vi "Store Calibration Coefficients.vi"(0 "Calibration Coefficients":T1[](array[typedef]) {"Elapsed Time" format="%<%H:%M:%S>t"; "zero_utc" format="%x"; "cal_utc" format="%x"; "Pump Flow Rate" format="%0d"; "Number of Zeroes" format="%0d"; "V2C" format="%0d"; "C2V" format="%0d"; "duration" format="%<%H:%M:%S>t"; "DAC" format="%03x"; "mI" format="%.3g"; "V_(RA,15mA)" format="%0.4f"; "V_(RA,5mA)" format="%0.4f"; "Chamber Temp" format="%.1f"; "Humidity" format="%.1f"}, 1 "Zero_Humidity":dbl format="%.2f", 2 "Zero_Temperature":dbl format="%.2f", 3 "supporting caldata":string[][](array[string])) -> ()   [LabVIEW 2016]
uses:
  Controls/Calibration Coefficients.ctl
  Miscellaneous/Globals.vi
  <vilib>/Utility/file.llb/Write To Spreadsheet File (string).vi
panel:
  in  "Logfile":path=path "calibration_log.csv"
  out "Spreadsheet Out":string[][](array[string])
  in  "Calfile":path=path "~last_calibration.csv"
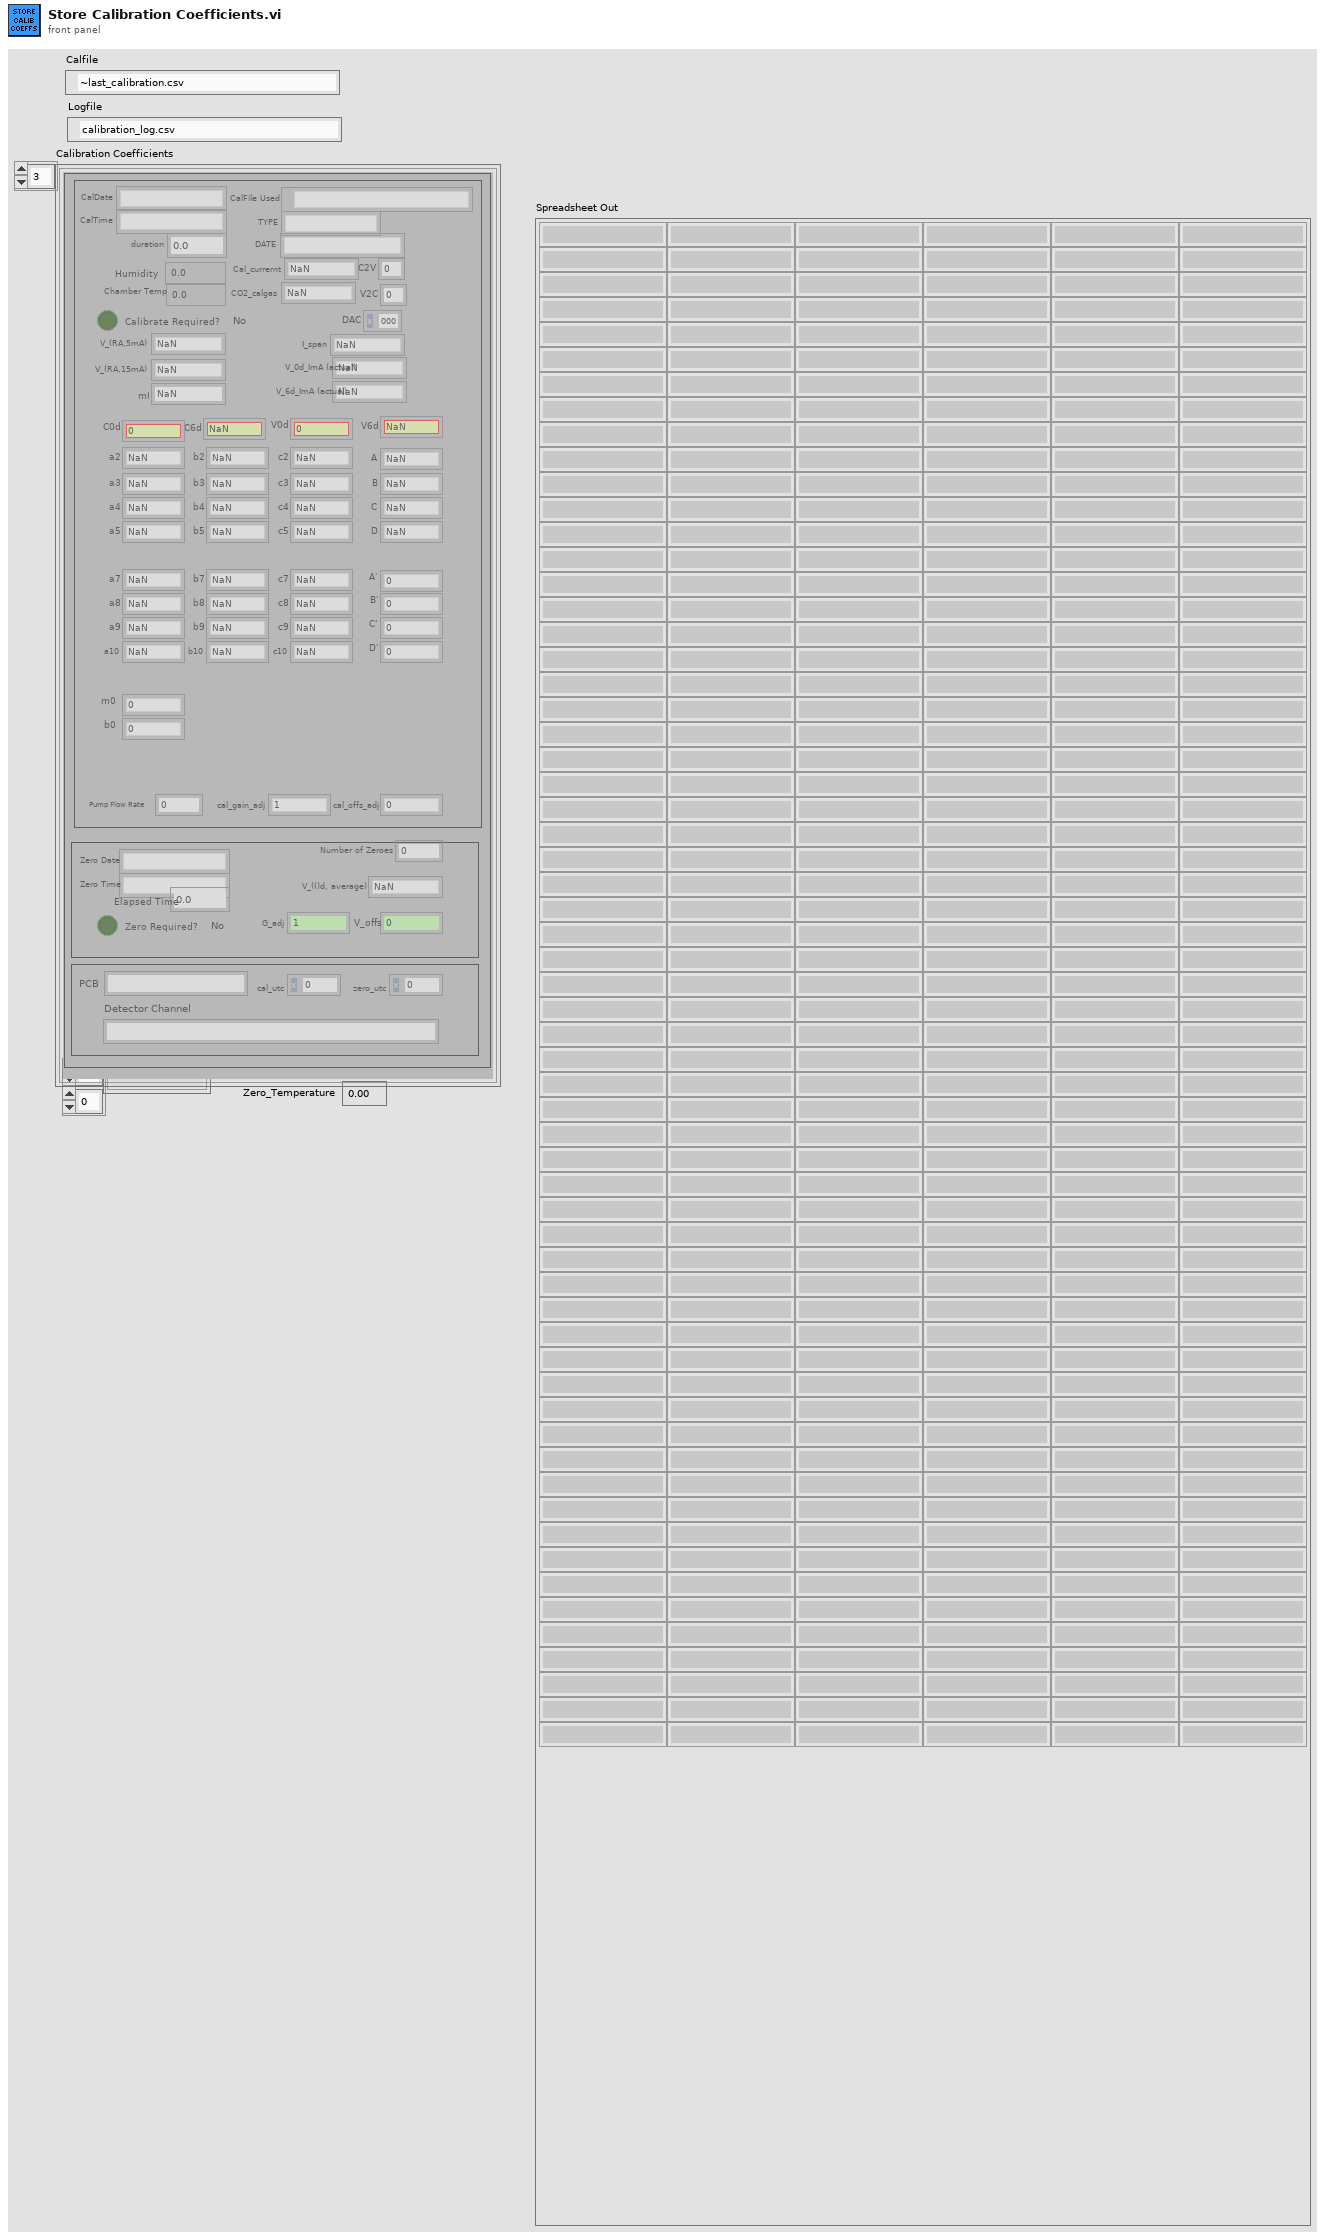
[diagram p1: front panel]
types:
  T1 = typedef "Calibration Coefficients.ctl" = cluster{"CalFile Used":path, "TYPE":string, "DATE":string, "Humidity":sgl, "Chamber Temp":dbl, "CO2_calgas":dbl, "V_(RA,5mA)":dbl, "V_(RA,15mA)":dbl, "mI":dbl, "V_0d_ImA (actual)":dbl, "V_6d_ImA (actual)":dbl, "I_span":dbl, "DAC":u16, "A":dbl, "B":dbl, "C":dbl, "D":dbl, "V6d":dbl, "A'":dbl, "B'":dbl, "C'":dbl, "D'":dbl, "V0d":dbl, "CalDate":string, "CalTime":string, "duration":dbl, "Detector Channel":string, "a2":dbl, "a3":dbl, "a4":dbl, "a5":dbl, "b2":dbl, "c2":dbl, "b3":dbl, "c3":dbl, "b4":dbl, "c4":dbl, "b5":dbl, "c5":dbl, "a7":dbl, "a8":dbl, "a9":dbl, "a10":dbl, "b7":dbl, "b8":dbl, "b9":dbl, "b10":dbl, "c7":dbl, "c8":dbl, "c9":dbl, "c10":dbl, "cal_offs_adj":dbl, "cal_gain_adj":dbl, "C6d":dbl, "C0d":dbl, "Cal_currernt":dbl, "C2V":u16, "V2C":u16, "Zero Date":string, "Zero Time":string, "Number of Zeroes":u16, "V_(()d, average)":dbl, "V_offs ":dbl, "G_adj":dbl, "Pump Flow Rate":u16, "Zero Required? ":bool, "Calibrate Required?":bool, "cal_utc":dbl, "zero_utc":dbl, "Elapsed Time":dbl, "PCB":string, "m0":dbl, "b0":dbl}
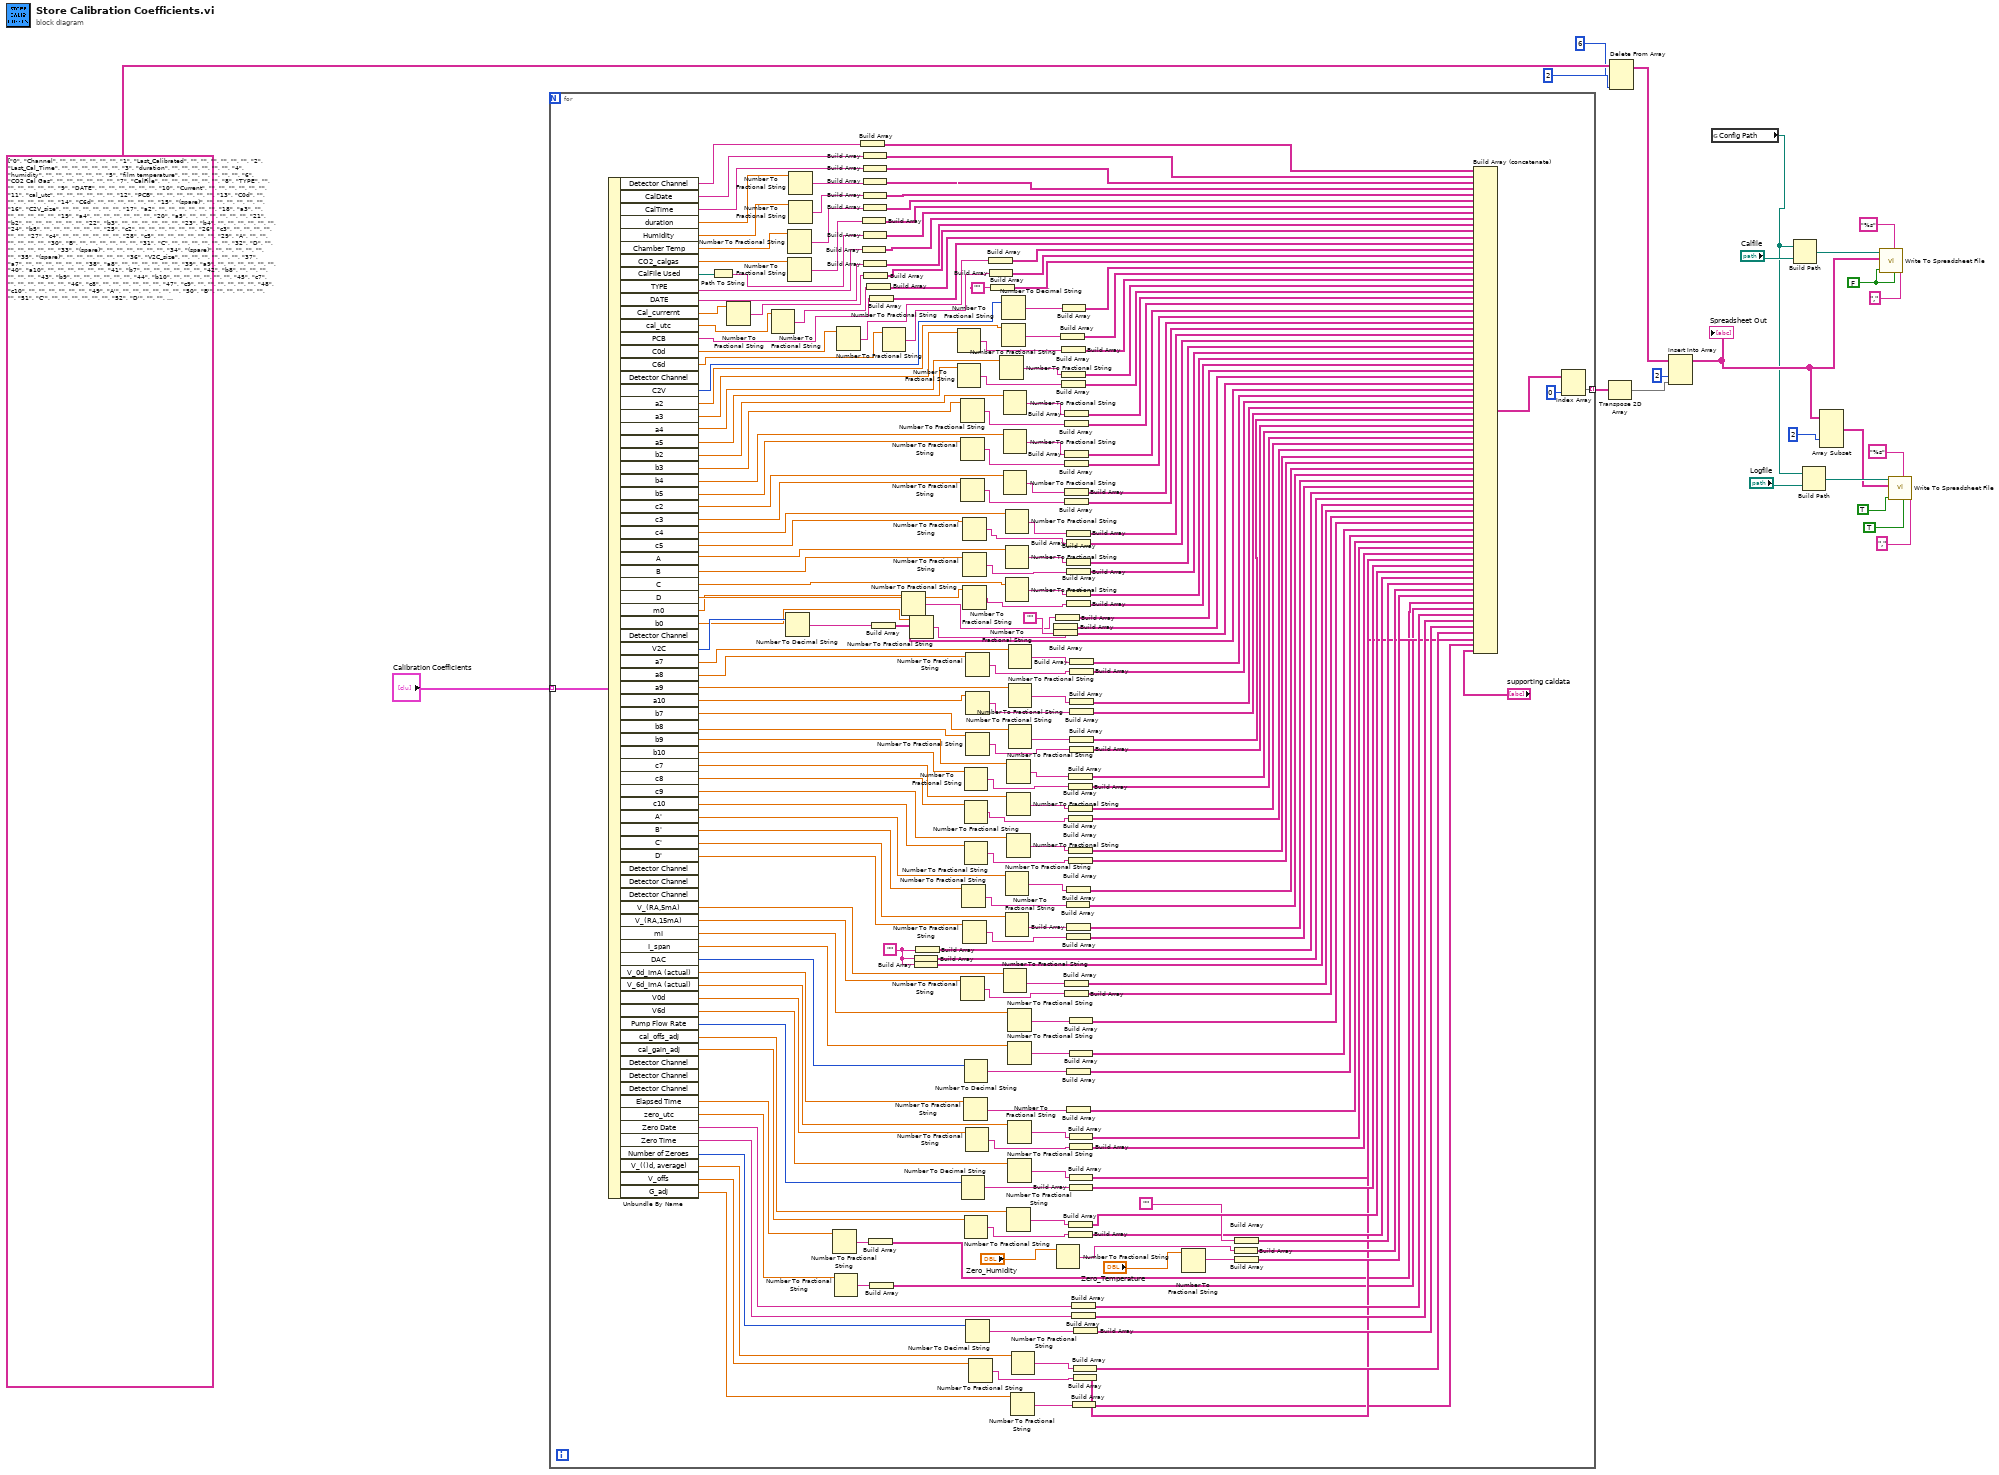
[diagram p0: block diagram]
diagram:
  w20 = FALSE ("transpose (no:F)")
  n1 = for {
    tunnel: [w166] -> w8 mode=indexing
    tunnel: "Calibration Coefficients" -> [w50] mode=indexing
    w87 = ""
    n2 = Unbundle By Name(w50) -> ("Detector Channel"=w55:string, "CalDate"=w249:string, "CalTime"=w248:string, "duration"=w246:dbl, "Humidity"=w163:sgl, "Chamber Temp"=w162:dbl, "CO2_calgas"=w157:dbl, "CalFile Used"=w155:path, "TYPE"=w153:string, "DATE"=w154:string, "Cal_currernt"=w44:dbl, "cal_utc"=w30:dbl, "PCB"=w28:string, "C0d"=w40:dbl, "C6d"=w39:dbl, "C2V"=w147:u16, "a2"=w145:dbl, "a3"=w144:dbl, "a4"=w143:dbl, "a5"=w142:dbl, "b2"=w141:dbl, "b3"=w140:dbl, "b4"=w139:dbl, "b5"=w138:dbl, "c2"=w137:dbl, "c3"=w136:dbl, "c4"=w135:dbl, "c5"=w134:dbl, "A"=w133:dbl, "B"=w132:dbl, "C"=w131:dbl, "D"=w130:dbl, "m0"=w27:dbl, "b0"=w26:dbl, "V2C"=w121:u16, "a7"=w124:dbl, "a8"=w123:dbl, "a9"=w114:dbl, "a10"=w113:dbl, "b7"=w112:dbl, "b8"=w111:dbl, "b9"=w110:dbl, "b10"=w109:dbl, "c7"=w108:dbl, "c8"=w107:dbl, "c9"=w106:dbl, "c10"=w105:dbl, "A'"=w103:dbl, "B'"=w102:dbl, "C'"=w101:dbl, "D'"=w100:dbl, "V_(RA,5mA)"=w99:dbl, "V_(RA,15mA)"=w98:dbl, "mI"=w97:dbl, "I_span"=w96:dbl, "DAC"=w90:u16, "V_0d_ImA (actual)"=w95:dbl, "V_6d_ImA (actual)"=w93:dbl, "V0d"=w92:dbl, "V6d"=w91:dbl, "Pump Flow Rate"=w89:u16, "cal_offs_adj"=w79:dbl, "cal_gain_adj"=w78:dbl, "Elapsed Time"=w42:dbl, "zero_utc"=w45:dbl, "Zero Date"=w71:string, "Zero Time"=w70:string, "Number of Zeroes"=w73:u16, "V_(()d, average)"=w68:dbl, "V_offs"=w67:dbl, "G_adj"=w66:dbl)  [unwired: 8 out]
    n3 = Path To String(path=w155) -> (string=w152:string)
    n4 = Number To Fractional String(number=w44) -> (F-format string=w31:string)  [unwired: 3 in]
    n5 = Number To Fractional String(number=w30) -> (F-format string=w29:string)  [unwired: 3 in]
    n6 = Number To Decimal String(number=w121) -> (decimal integer string=w122:string)  [unwired: 1 in]
    n7 = Number To Fractional String(number=w162) -> (F-format string=w160:string)  [unwired: 3 in]
    n8 = Number To Fractional String(number=w157) -> (F-format string=w156:string)  [unwired: 3 in]
    n9 = Number To Fractional String(number=w246) -> (F-format string=w245:string)  [unwired: 3 in]
    n10 = Number To Fractional String(number=w163) -> (F-format string=w161:string)  [unwired: 3 in]
    n11 = Number To Fractional String(number=w42) -> (F-format string=w43:string)  [unwired: 3 in]
    n12 = Number To Fractional String(number=w45) -> (F-format string=w47:string)  [unwired: 3 in]
    n13 = Number To Fractional String(number=w40) -> (F-format string=w37:string)  [unwired: 3 in]
    n14 = Build Array(w55) -> (w54:string[])
    n15 = Build Array(w156) -> (w151:string[])
    n16 = Build Array(w153) -> (w149:string[])
    n17 = Build Array(w249) -> (w247:string[])
    n18 = Build Array(w248) -> (w53:string[])
    n19 = Build Array(w245) -> (w164:string[])
    n20 = Build Array(w161) -> (w159:string[])
    n21 = Build Array(w160) -> (w158:string[])
    n22 = Build Array(w152) -> (w150:string[])
    n23 = Build Array(w154) -> (w148:string[])
    n24 = Build Array(w31) -> (w129:string[])
    n25 = Build Array(w29) -> (w48:string[])
    n26 = Build Array(w43) -> (w41:string[])
    n27 = Build Array(w28) -> (w128:string[])
    n28 = Build Array(w47) -> (w46:string[])
    n29 = Build Array(w122) -> (w119:string[])
    n30 = Number To Fractional String(number=w39) -> (F-format string=w38:string)  [unwired: 3 in]
    n31 = Number To Fractional String(number=w27) -> (F-format string=w25:string)  [unwired: 3 in]
    n32 = Number To Fractional String(number=w26) -> (F-format string=w24:string)  [unwired: 3 in]
    n33 = Build Array(w87) -> (w85:string[])
    n34 = Build Array(w87) -> (w84:string[])
    n35 = Build Array(w87) -> (w86:string[])
    n36 = Number To Fractional String(number=w144) -> (F-format string=w233:string)  [unwired: 3 in]
    n37 = Number To Fractional String(number=w142) -> (F-format string=w232:string)  [unwired: 3 in]
    n38 = Number To Fractional String(number=w140) -> (F-format string=w231:string)  [unwired: 3 in]
    n39 = Number To Fractional String(number=w138) -> (F-format string=w223:string)  [unwired: 3 in]
    n40 = Number To Fractional String(number=w136) -> (F-format string=w230:string)  [unwired: 3 in]
    n41 = Number To Fractional String(number=w98) -> (F-format string=w210:string)  [unwired: 3 in]
    n42 = Number To Decimal String(number=w89) -> (decimal integer string=w82:string)  [unwired: 1 in]
    n43 = Number To Fractional String(number=w102) -> (F-format string=w104:string)  [unwired: 3 in]
    n44 = Number To Fractional String(number=w134) -> (F-format string=w229:string)  [unwired: 3 in]
    n45 = Number To Fractional String(number=w132) -> (F-format string=w228:string)  [unwired: 3 in]
    n46 = Number To Fractional String(number=w130) -> (F-format string=w227:string)  [unwired: 3 in]
    n47 = Number To Fractional String(number=w100) -> (F-format string=w222:string)  [unwired: 3 in]
    n48 = Number To Fractional String(number=w95) -> (F-format string=w88:string)  [unwired: 3 in]
    n49 = Number To Fractional String(number=w109) -> (F-format string=w219:string)  [unwired: 3 in]
    n50 = Number To Fractional String(number=w107) -> (F-format string=w220:string)  [unwired: 3 in]
    n51 = Number To Fractional String(number=w105) -> (F-format string=w221:string)  [unwired: 3 in]
    n52 = Number To Decimal String(number=w90) -> (decimal integer string=w94:string)  [unwired: 1 in]
    n53 = Number To Fractional String(number=w78) -> (F-format string=w80:string)  [unwired: 3 in]
    n54 = Number To Fractional String(number=w92) -> (F-format string=w211:string)  [unwired: 3 in]
    n55 = Number To Fractional String(number=w123) -> (F-format string=w226:string)  [unwired: 3 in]
    n56 = Number To Fractional String(number=w113) -> (F-format string=w225:string)  [unwired: 3 in]
    n57 = Number To Fractional String(number=w111) -> (F-format string=w224:string)  [unwired: 3 in]
    n58 = Number To Decimal String(number=w73) -> (decimal integer string=w75:string)  [unwired: 1 in]
    n59 = Number To Fractional String(number=w67) -> (F-format string=w77:string)  [unwired: 3 in]
    n60 = Build Array(w37) -> (w127:string[])
    n61 = Build Array(w38) -> (w126:string[])
    n62 = Build Array("") -> (w125:string[])
    n63 = Number To Fractional String(number=w143) -> (F-format string=w234:string)  [unwired: 3 in]
    n64 = Number To Decimal String(number=w147) -> (decimal integer string=w244:string)  [unwired: 1 in]
    n65 = Number To Fractional String(number=w145) -> (F-format string=w146:string)  [unwired: 3 in]
    n66 = Number To Fractional String(number=w141) -> (F-format string=w235:string)  [unwired: 3 in]
    n67 = Number To Fractional String(number=w139) -> (F-format string=w236:string)  [unwired: 3 in]
    n68 = Number To Fractional String(number=w137) -> (F-format string=w237:string)  [unwired: 3 in]
    n69 = Number To Fractional String(number=w99) -> (F-format string=w209:string)  [unwired: 3 in]
    n70 = Number To Fractional String(number=w135) -> (F-format string=w238:string)  [unwired: 3 in]
    n71 = Number To Fractional String(number=w133) -> (F-format string=w239:string)  [unwired: 3 in]
    n72 = Number To Fractional String(number=w131) -> (F-format string=w240:string)  [unwired: 3 in]
    n73 = Number To Fractional String(number=w103) -> (F-format string=w215:string)  [unwired: 3 in]
    n74 = Number To Fractional String(number=w101) -> (F-format string=w216:string)  [unwired: 3 in]
    n75 = Number To Fractional String(number=w110) -> (F-format string=w185:string)  [unwired: 3 in]
    n76 = Number To Fractional String(number=w108) -> (F-format string=w218:string)  [unwired: 3 in]
    n77 = Number To Fractional String(number=w106) -> (F-format string=w217:string)  [unwired: 3 in]
    n78 = Number To Fractional String(number=w79) -> (F-format string=w81:string)  [unwired: 3 in]
    n79 = Number To Fractional String(number=w97) -> (F-format string=w176:string)  [unwired: 3 in]
    n80 = Number To Fractional String(number=w96) -> (F-format string=w212:string)  [unwired: 3 in]
    n81 = Number To Fractional String(number=w93) -> (F-format string=w213:string)  [unwired: 3 in]
    n82 = Number To Fractional String(number=w91) -> (F-format string=w214:string)  [unwired: 3 in]
    n83 = Number To Fractional String(number=w124) -> (F-format string=w241:string)  [unwired: 3 in]
    n84 = Number To Fractional String(number=w114) -> (F-format string=w243:string)  [unwired: 3 in]
    n85 = Number To Fractional String(number=w112) -> (F-format string=w242:string)  [unwired: 3 in]
    n86 = Number To Fractional String(number=w66) -> (F-format string=w74:string)  [unwired: 3 in]
    n87 = Number To Fractional String(number=w68) -> (F-format string=w76:string)  [unwired: 3 in]
    n88 = Build Array(w24) -> (w116:string[])
    n89 = Build Array("") -> (w117:string[])
    n90 = Build Array(w25) -> (w115:string[])
    n91 = Number To Fractional String(number="Zero_Humidity") -> (F-format string=w35:string)  [unwired: 3 in]
    n92 = Build Array(w146) -> (w120:string[])
    n93 = Build Array(w233) -> (w208:string[])
    n94 = Build Array(w234) -> (w207:string[])
    n95 = Build Array(w232) -> (w206:string[])
    n96 = Build Array(w244) -> (w52:string[])
    n97 = Build Array(w235) -> (w205:string[])
    n98 = Build Array(w231) -> (w204:string[])
    n99 = Build Array(w236) -> (w203:string[])
    n100 = Build Array(w223) -> (w202:string[])
    n101 = Build Array(w237) -> (w201:string[])
    n102 = Build Array(w230) -> (w200:string[])
    n103 = Build Array(w209) -> (w177:string[])
    n104 = Build Array(w210) -> (w175:string[])
    n105 = Build Array(w104) -> (w51:string[])
    n106 = Build Array(w238) -> (w199:string[])
    n107 = Build Array(w229) -> (w198:string[])
    n108 = Build Array(w239) -> (w197:string[])
    n109 = Build Array(w228) -> (w196:string[])
    n110 = Build Array(w240) -> (w195:string[])
    n111 = Build Array(w227) -> (w194:string[])
    n112 = Build Array(w215) -> (w180:string[])
    n113 = Build Array(w216) -> (w179:string[])
    n114 = Build Array(w222) -> (w178:string[])
    n115 = Build Array(w94) -> (w83:string[])
    n116 = Build Array(w88) -> (w172:string[])
    n117 = Build Array(w185) -> (w187:string[])
    n118 = Build Array(w219) -> (w186:string[])
    n119 = Build Array(w218) -> (w184:string[])
    n120 = Build Array(w220) -> (w183:string[])
    n121 = Build Array(w217) -> (w182:string[])
    n122 = Build Array(w221) -> (w181:string[])
    n123 = Build Array(w81) -> (w72:string[])
    n124 = Build Array(w80) -> (w65:string[])
    n125 = Build Array(w176) -> (w174:string[])
    n126 = Build Array(w212) -> (w173:string[])
    n127 = Build Array(w213) -> (w171:string[])
    n128 = Build Array(w211) -> (w170:string[])
    n129 = Build Array(w214) -> (w169:string[])
    n130 = Build Array(w82) -> (w168:string[])
    n131 = Build Array(w241) -> (w193:string[])
    n132 = Build Array(w226) -> (w192:string[])
    n133 = Build Array(w243) -> (w191:string[])
    n134 = Build Array(w225) -> (w190:string[])
    n135 = Build Array(w242) -> (w189:string[])
    n136 = Build Array(w224) -> (w188:string[])
    n137 = Build Array(w71) -> (w61:string[])
    n138 = Build Array(w70) -> (w60:string[])
    n139 = Build Array(w74) -> (w56:string[])
    n140 = Build Array(w76) -> (w58:string[])
    n141 = Build Array(w77) -> (w57:string[])
    n142 = Build Array(w75) -> (w59:string[])
    n143 = Number To Fractional String(number="Zero_Temperature") -> (F-format string=w34:string)  [unwired: 3 in]
    n144 = Build Array(w35) -> (w63:string[])
    n145 = Build Array("") -> (w64:string[])
    n146 = Build Array(w34) -> (w62:string[])
    n147 = Build Array (concatenate)(w54, w247, w53, w164, w159, w158, w151, w150, w149, w148, w129, w48, w128, w127, w126, w125, w52, w120, w208, w207, w206, w205, w204, w203, w202, w201, w200, w199, w198, w197, w196, w195, w194, w115, w116, w117, w119, w193, w192, w191, w190, w189, w188, w187, w186, w184, w183, w182, w181, w180, w51, w179, w178, w86, w85, w84, w177, w175, w174, w173, w83, w172, w171, w170, w169, w168, w72, w65, w64, w63, w62, w41, w46, w61, w60, w59, w58, w57, w56, "supporting caldata") -> (w167:string[][])
    n148 = Index Array(array=w167, index (col)=0 ("disabled index (col)")) -> (element=w166:string[])  [unwired: 1 in]
  }
  n149 = Transpose 2D Array(2D array=w8) -> (transposed array=w4:string[][])
  n150 = Delete From Array(array=string[][] [["0", "Channel", "", "", "", "", "", ""], ["1", "Last_Calibrated", "", "", "", "", "", ""], ["2", "Last_Cal_Time", "", "", "", "", "", ""], ["3", "duration", "", "", "", "", "", ""], ["4", "humidity", "", "", "", "", "", ""], ["5", "film temperature", "", "", "", "", "", ""], ["6", "CO2 Cal Gas", "", "", "", "", "", ""], ["7", "CalFile", "", "", "", "", "", ""], ["8", "TYPE", "", "", "", "", "", ""], ["9", "DATE", "", "", "", "", "", ""], ["10", "Current", "", "", "", "", "", ""], ["11", "cal_utc", "", "", "", "", "", ""], ["12", "PCB", "", "", "", "", "", ""], ["13", "C0d", "", "", "", "", "", ""], ["14", "C6d", "", "", "", "", "", ""], ["15", "(spare)", "", "", "", "", "", ""], ["16", "C2V_size", "", "", "", "", "", ""], ["17", "a2", "", "", "", "", "", ""], ["18", "a3", "", "", "", "", "", ""], ["19", "a4", "", "", "", "", "", ""], ["20", "a5", "", "", "", "", "", ""], ["21", "b2", "", "", "", "", "", ""], ["22", "b3", "", "", "", "", "", ""], ["23", "b4", "", "", "", "", "", ""], ["24", "b5", "", "", "", "", "", ""], ["25", "c2", "", "", "", "", "", ""], ["26", "c3", "", "", "", "", "", ""], ["27", "c4", "", "", "", "", "", ""], ["28", "c5", "", "", "", "", "", ""], ["29", "A", "", "", "", "", "", ""], ["30", "B", "", "", "", "", "", ""], ["31", "C", "", "", "", "", "", ""], ["32", "D", "", "", "", "", "", ""], ["33", "(spare)", "", "", "", "", "", ""], ["34", "(spare)", "", "", "", "", "", ""], ["35", "(spare)", "", "", "", "", "", ""], ["36", "V2C_size", "", "", "", "", "", ""], ["37", "a7", "", "", "", "", "", ""], ["38", "a8", "", "", "", "", "", ""], ["39", "a9", "", "", "", "", "", ""], ["40", "a10", "", "", "", "", "", ""], ["41", "b7", "", "", "", "", "", ""], ["42", "b8", "", "", "", "", "", ""], ["43", "b9", "", "", "", "", "", ""], ["44", "b10", "", "", "", "", "", ""], ["45", "c7", "", "", "", "", "", ""], ["46", "c8", "", "", "", "", "", ""], ["47", "c9", "", "", "", "", "", ""], ["48", "c10", "", "", "", "", "", ""], ["49", "A'", "", "", "", "", "", ""], ["50", "B'", "", "", "", "", "", ""], ["51", "C'", "", "", "", "", "", ""], ["52", "D'", "", "", "", "", "", ""], ["53", "(spare)", "", "", "", "", "", ""], ["54", "(spare)", "", "", "", "", "", ""], ["55", "(spare)", "", "", "", "", "", ""], ["56", "V_RA_5", "", "", "", "", "", ""], ["57", "V_RA_15", "", "", "", "", "", ""], ["58", "mI", "", "", "", "", "", ""], ["59", "I_span", "", "", "", "", "", ""], ["60", "DAC", "", "", "", "", "", ""], ["61", "V_0d_ImA (actual)", "", "", "", "", "", ""], ["62", "V_6d_ImA (actual)", "", "", "", "", "", ""], ["63", "V_0d_target", "", "", "", "", "", ""], ["64", "V_6d_target", "", "", "", "", "", ""], ["65", "Pump_Flow_rate", "", "", "", "", "", ""], ["66", "Cal_Offset_adj", "", "", "", "", "", ""], ["67", "Cal_Gain_adj", "", "", "", "", "", ""], ["68", "(spare)", "", "", "", "", "", ""], ["69", "last_zero_humidity", "", "", "", "", "", ""], ["70", "last_zero_humidity", "", "", "", "", "", ""], ["71", "Time Monitoring since last zero", "", "", "", "", "", ""], ["72", "zero_utc", "", "", "", "", "", ""], ["73", "Last_Zero'd", "", "", "", "", "", ""], ["74", "Last_Zero_Time", "", "", "", "", "", ""], ["75", "Number_of_Zeros", "", "", "", "", "", ""], ["76", "V_0d_average", "", "", "", "", "", ""], ["77", "V_Offset_adj", "", "", "", "", "", ""], ["78", "V_Gain_adj", "", "", "", "", "", ""], ["79", "Software Rev", "", "", "", "", "", ""], ["80", "Sample Descriptor", "", "", "", "", "", ""], ["81", "Chamber", "", "", "", "", "", ""], ["82", "Operator", "", "", "", "", "", ""], ["83", "Notes", "", "", "", "", "", ""], ["84", "END", "", "", "", "", "", ""]] ("Spreadsheet Template"), length=6, index (col)=2 ("index (row)")) -> (array with subset deleted=w5:string[][])  [unwired: 1 in, 1 out]
  n151 = Insert Into Array(array=w5, index (col)=2 ("disabled index (col)"), new element=w4) -> (w2:string[][])  [unwired: 1 in]
  "Spreadsheet Out" <- w2
  n152 = global read "Globals.vi" "Config Path"() -> (w1:path)
  n153 = Build Path(base path=w1, name or relative path="Calfile") -> (appended path=w22:path)
  n154 = Build Path(base path=w1, name or relative path="Logfile") -> (appended path=w14:path)
  n155 = Array Subset(array=w2, index (col)=2 ("index (row)")) -> (w11:string[][])  [unwired: 3 in]
  n156 = call-poly <vilib>:"Write To Spreadsheet File.vi"("delimiter (\\t)"="," ("delimiter (\\t)"), "transpose? (no:F)"=w20, "format (%s)"="%s" ("format (%d)"), "append to file? (new file:F)"=w20, "2D data"=w2, "file path (dialog if empty)"=w22) -> ()  [unwired: 2 in, 1 out]
  n157 = call-poly <vilib>:"Write To Spreadsheet File.vi"("delimiter (\\t)"="," ("delimiter (\\t)"), "transpose? (no:F)"=TRUE ("transpose (no:F)"), "format (%s)"="%s" ("format (%d)"), "append to file? (new file:F)"=TRUE ("transpose (no:F)"), "2D data"=w11, "file path (dialog if empty)"=w14) -> ()  [unwired: 2 in, 1 out]
